vi "time_formatter.vi"(11 "time (ms)":dbl) -> (2 "time (sec)":dbl, 3 "Elasped Time (HH:MM:SS)":string caption="Result")   [LabVIEW 2021]
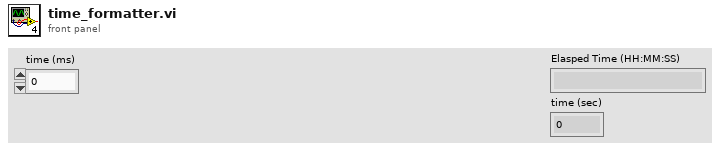
[diagram p1: front panel]
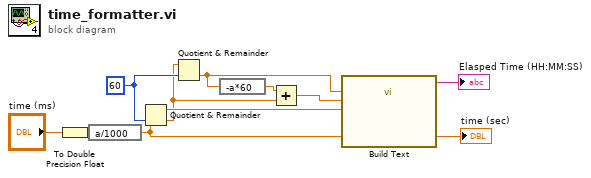
[diagram p0: block diagram]
diagram:
  w8 = 60
  n1 = To Double Precision Float(number="time (ms)") -> (double precision float=w7:dbl)
  n2 = expression code="a/1000"(w7) -> (w9:dbl)
  "time (sec)" <- w9
  n3 = Quotient & Remainder(x=w9, y=w8) -> (x-y*floor(x/y)=w10:dbl, floor(x/y)=w3:dbl)
  n4 = Quotient & Remainder(x=w3, y=w8) -> (floor(x/y)=w5:dbl)  [unwired: 1 out]
  n5 = expression code="-a*60"(w5) -> (w4:dbl)
  n6 = Add(x=w4, y=w3) -> (x+y=w2:dbl)
  n7 = call "Build Text"("hours"=w5, "minutes"=w2, "seconds"=w10) -> ("Result"=→"Elasped Time (HH:MM:SS)":string)  [unwired: 11 in, 1 out]
